vi "Resolve IP.vi"(7 "IP Target (Local)":T1, 8 "error in (no error)":errorcluster, 11 "IP Resolver in":refnum<class "IP Resolver.lvclass">) -> (0 "error out":errorcluster, 2 "U32 Address":u32 format="%08x", 3 "IP Resolver out":refnum<class "IP Resolver.lvclass">)   [LabVIEW 2020, in "Vecto.lvlib" / "IP Resolver.lvclass"]
uses:
  IP Resolver.lvclass
  IP Resolver.lvclass/IP Resolver.ctl
  1e9f654b-1a30-470d-964a-3fedf4ea8f42.vi
  IP Target.ctl
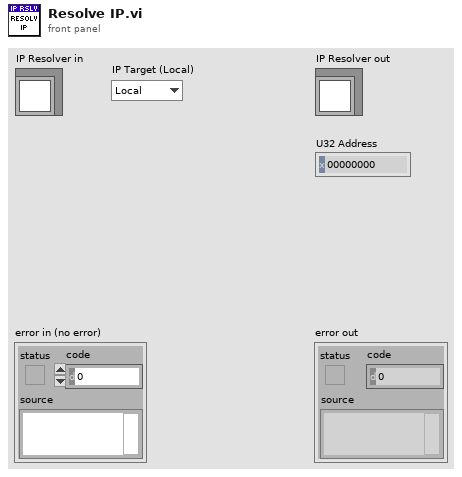
[diagram p1: front panel]
types:
  T1 = typedef "Vecto.lvlib/IP Resolver.lvclass/IP Target.ctl" = enum16{"Local", "External"}
  T2 = typedef "Vecto.lvlib/IP Resolver.lvclass/Bind Info.ctl" = cluster{"Type":T3, "Binding":string, "Subnet Bits":i32}
  T3 = typedef "Vecto.lvlib/IP Resolver.lvclass/Address Type.ctl" = enum16{"Unknown", "Specific", "Subnet", "Any"}
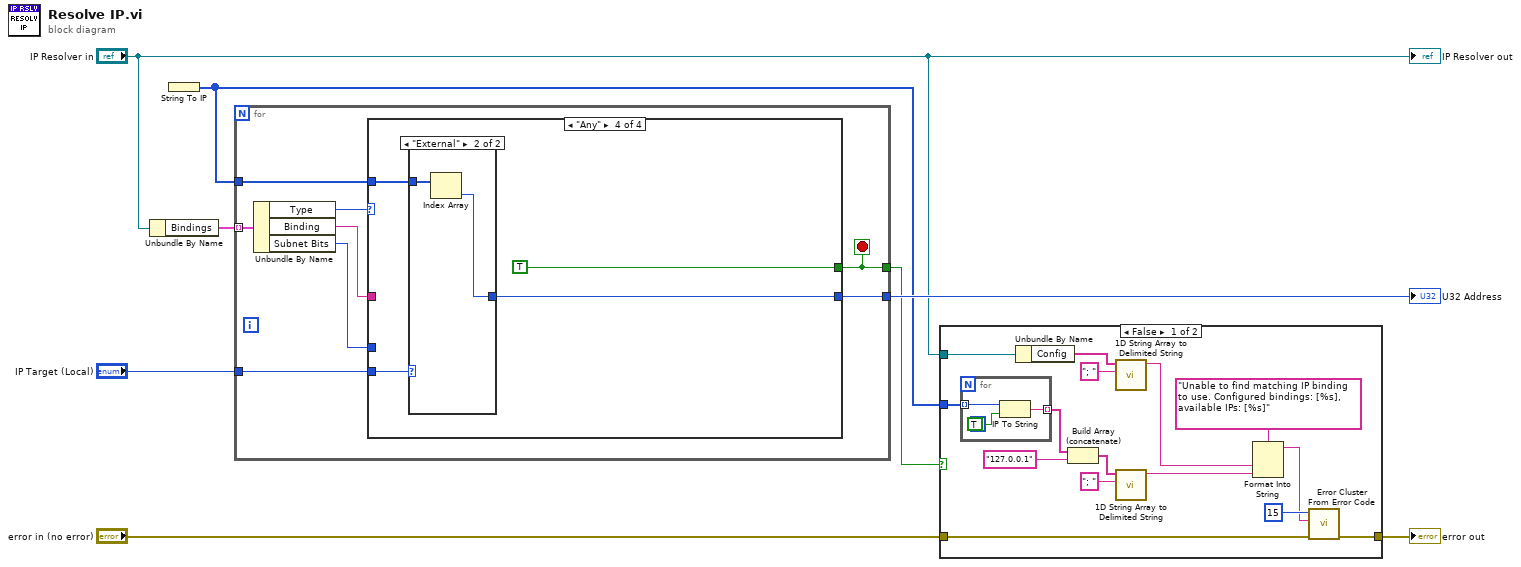
[diagram p0: block diagram]
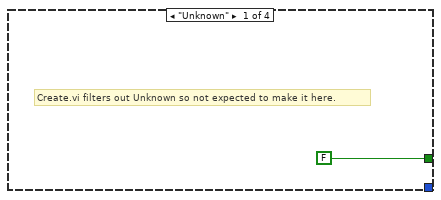
[diagram p3: hidden frame]
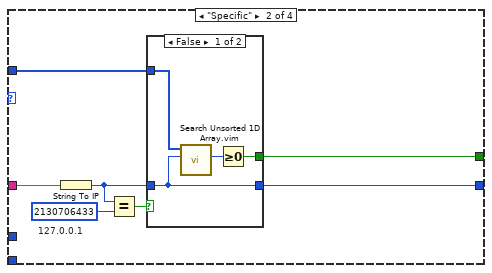
[diagram p4: hidden frame]
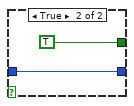
[diagram p5: hidden frame]
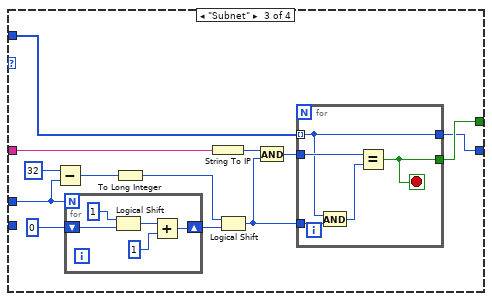
[diagram p6: hidden frame]
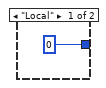
[diagram p7: hidden frame]
diagram:
  n1 = Unbundle By Name("IP Resolver in") -> ("Bindings"=w8:T2[])
  n2 = String To IP() -> (0:w2:u32[])  [unwired: 1 in]
  n3 = for {
    tunnel: w8 -> [w16] mode=indexing
    tunnel: "IP Target (Local)" -> [w11]
    tunnel: w2 -> [w12]
    tunnel: [w10] -> w4
    tunnel: [w9] -> w6
    stop <- w10 stop-if-true
    n4 = Unbundle By Name(w16) -> ("Type"=w15:T3, "Binding"=w14:string, "Subnet Bits"=w13:i32)
    n5 = case shown="\"Any\"" w15 {
      tunnel: w14 -> [_ w23 w35 _]
      tunnel: [_ w24 w31 w57] -> w9
      tunnel: w13 -> [_ _ w34 _]
      tunnel: w12 -> [_ w19 w33 w55]
      tunnel: [FALSE w18 w32 TRUE] -> w10
      tunnel: w11 -> [_ _ _ w56]
      frame "Unknown" {
        # "Create.vi filters out Unknown so not expected to make it here."
      }
      frame "Specific" {
        w21 = u32 2130706433  # 127.0.0.1
        n6 = String To IP(1:w23) -> (0:w22:u32)
        n7 = Equal?(x=w22, y=w21) -> (x = y?=w20:bool)
        n8 = case shown="False" w20 {
          tunnel: [w25 w30] -> w24
          tunnel: w22 -> [w25 w30]
          tunnel: w19 -> [w28 _]
          tunnel: [w26 TRUE] -> w18
          frame False {
            n9 = call "Search Unsorted 1D Array.vim"("element"=w25, "unsorted 1D array"=w28) -> ("index of element"=w27:i32)  [unwired: 9 in]
            n10 = Greater Or Equal To 0?(x=w27) -> (x >= 0?=w26:bool)
          }
          frame True {
          }
        }
      }
      frame "Subnet" {
        n11 = Subtract(x=32, y=w34) -> (x-y=w41:i32)
        n12 = for {
          N: w34 -> [_]
          shift-right: [w49] -> w40
          shift-left: u32 0 -> [w53]
          n13 = Logical Shift(y=i16 1, x=w53) -> (x << y=w51:u32)
          n14 = Add(x=w51, y=u32 1) -> (x+y=w49:u32)
        }
        n15 = To Long Integer(number=w41) -> (32bit integer=w39:i32)
        n16 = String To IP(1:w35) -> (0:w38:u32)
        n17 = Logical Shift(y=w39, x=w40) -> (x << y=w36:u32)
        n18 = And(x=w38, y=w36) -> (x .and. y?=w37:u32)
        n19 = for {
          tunnel: w37 -> [w47]
          tunnel: w33 -> [w45] mode=indexing
          tunnel: w36 -> [w48]
          tunnel: [w45] -> w31
          tunnel: [w44] -> w32
          stop <- w44 stop-if-true
          n20 = And(x=w45, y=w48) -> (x .and. y?=w46:u32)
          n21 = Equal?(x=w47, y=w46) -> (x = y?=w44:bool)
        }
      }
      frame "Any" {
        n22 = case shown="\"External\"" w56 {
          tunnel: [u32 0 w59] -> w57
          tunnel: w55 -> [_ w60]
          frame "Local" {
          }
          frame "External" {
            n23 = Index Array(array=w60) -> (element=w59:u32)  [unwired: 1 in]
          }
        }
      }
    }
  }
  "U32 Address" <- w6
  n24 = case shown="False" w4 {
    tunnel: "error in (no error)" -> [w64 w79]
    tunnel: [w63 w79] -> w3
    tunnel: w2 -> [w75 _]
    tunnel: "IP Resolver in" -> [w70 _]
    frame False {
      n25 = for {
        tunnel: w75 -> [w78] mode=indexing
        tunnel: [w76] -> w73 mode=indexing
        n26 = IP To String(1:TRUE ("dot notation? (F)"), 2:w78) -> (0:w76:string)
      }
      n27 = Unbundle By Name(w70) -> ("Config"=w68:string[])
      n28 = Build Array (concatenate)(w73, "127.0.0.1") -> (w72:string[])
      n29 = call <vilib>:"1D String Array to Delimited String.vi"("delimiter"="; ", "string array"=w68) -> ("delimited string"=w66:string)  [unwired: 9 in]
      n30 = call <vilib>:"1D String Array to Delimited String.vi"("delimiter"="; ", "string array"=w72) -> ("delimited string"=w65:string)  [unwired: 9 in]
      n31 = Format Into String(format string="Unable to find matching IP binding to use. Configured bindings: [%s], available IPs: [%s]", w66, w65) -> (resulting string=w61:string)  [unwired: 2 in, 1 out]
      n32 = call <vilib>:"Error Cluster From Error Code.vi"("error in (no error)"=w64, "error message (\"\")"=w61, "error code (0)"=15) -> ("error out"=w63:errorcluster)  [unwired: 6 in]
    }
    frame True {
    }
  }
  "error out" <- w3
  "IP Resolver out" <- "IP Resolver in"
